vi "Setup Viewers speed graph during runtime.vi"(8 "error in (no error)":errorcluster, 11 "Frame number":i32) -> (0 "error out":errorcluster)   [LabVIEW 2013]
uses:
  Functional Imaging Viewer/Typedefs/Get-Set-Clear Control.ctl
  Globals/gl_Time series viewer globals.vi
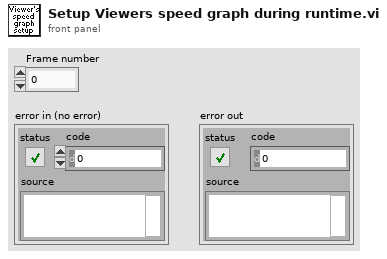
[diagram p1: front panel]
types:
  T1 = typedef "Get-Set-Clear Control.ctl" = enum16{"Get", "Set", "Clear"}
  T2 = typedef "Timelapse viewer refs.ctl" = cluster{"This VI":refnum<vi>, "AVI Mode ind":refnum<vi>, "Play":refnum<vi>, "Stop":refnum<vi>, "Back":refnum<vi>, "Scrollbar":refnum<vi>, "Video length info":refnum<vi>, "Expected speed values":refnum<vi>, "Intensity":refnum<vi>, "Path":refnum<vi>, "Selection sliders":refnum<vi>, "Speed Graph ref":refnum<vi>, "Frame rate set (fps)":refnum<vi>}
  T3 = typedef "Speed graph behaviour enum.ctl" = enum16{"Scrolling data", "Scrolling cursor"}
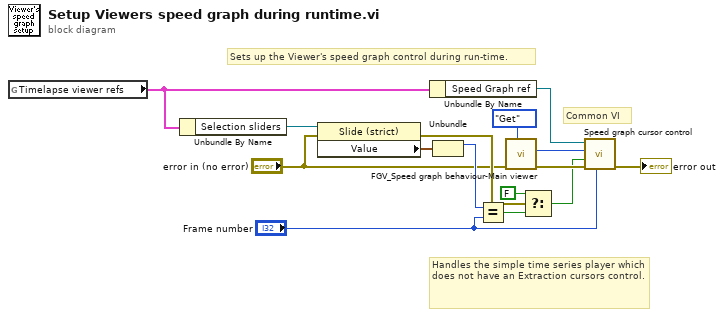
[diagram p0: block diagram]
diagram:
  # "Handles the simple time series player which does not have an Extraction cursors control."
  # "Sets up the Viewer's speed graph control during run-time."
  # "Common VI"
  n1 = global read "gl_Time series viewer globals.vi" "Timelapse viewer refs"() -> (w15:T2)
  n2 = Unbundle By Name(w15) -> ("Selection sliders"=w13:refnum<vi>)
  n3 = property on="Property Node" class="Slide (strict)"(reference=w13, error in="error in (no error)") -> (error out=w3:errorcluster, "Value"=w12:cluster{i32, i32})  [unwired: 1 out]
  n4 = Unbundle By Name(w15) -> ("Speed Graph ref"=w11:refnum<vi>)
  n5 = Unbundle(w12) -> (w14:i32)  [unwired: 1 out]
  n6 = Equal?(x=w14, y="Frame number") -> (x = y?=w5:bool)
  n7 = call "FGV_Speed graph behaviour-Main viewer.vi"("Function"=Get-Set-Clear_Control."Get", "error in (no error)"="error in (no error)") -> ("error out"=w7:errorcluster, "Speed graph behaviour"=w10:T3)  [unwired: 8 in]
  n8 = Select(t=FALSE, s=w3, f=w5) -> (s? t:f=w4:bool)
  n9 = call "Speed graph cursor control.vi"("Frame number"="Frame number", "error in (no error)"=w7, "Initial frame"=w4, "Speed graph behaviour"=w10, "Speed graph ref"=w11) -> ("error out"=→"error out":errorcluster)  [unwired: 6 in]
